vi "Write Position.vi"(8 "error in (no error)":errorcluster, 10 "Position":dbl, 11 "MoveAfterReference Msg in":refnum<class "MoveAfterReference Msg.lvclass">) -> (0 "error out":errorcluster, 3 "MoveAfterReference Msg out":refnum<class "MoveAfterReference Msg.lvclass">)   [LabVIEW 2015, in "CS++Motor.lvlib" / "MoveAfterReference Msg.lvclass"]
uses:
  MoveAfterReference Msg.lvclass
  MoveAfterReference Msg.lvclass/MoveAfterReference Msg.ctl
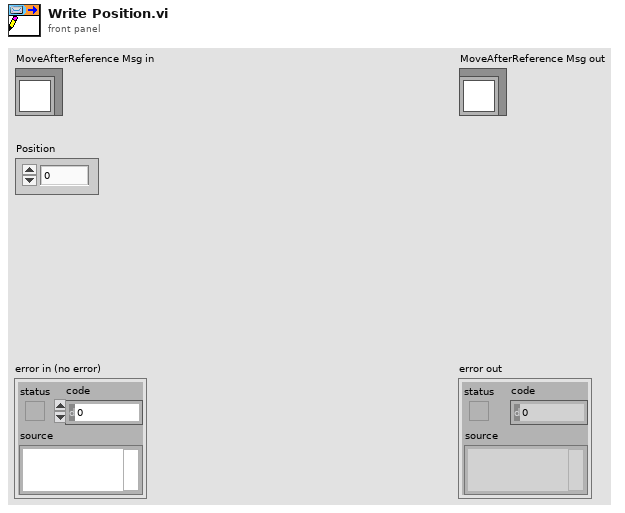
[diagram p1: front panel]
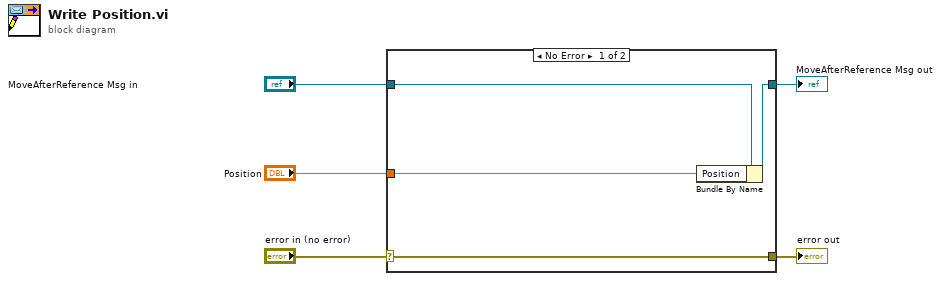
[diagram p0: block diagram]
diagram:
  n1 = case shown="No Error" "error in (no error)" {
    selector: "error in (no error)" -> [w9 w10]
    tunnel: [w9 w10] -> w4
    tunnel: [w7 w11] -> w2
    tunnel: "MoveAfterReference Msg in" -> [w8 w11]
    tunnel: "Position" -> [w6 _]
    frame No Error {
      n2 = Bundle By Name(cluster=w8, "Position"=w6) -> (w7:refnum<class "MoveAfterReference Msg.lvclass">)
    }
    frame Error {
    }
  }
  "error out" <- w4
  "MoveAfterReference Msg out" <- w2
